vi "Expt 6.vi"() -> ()   [LabVIEW 2020]
panel:
  out "x >= 0?":bool
  out "current time":timestamp
  out "Y":dbl
  in  "y":dbl
  in  "x":dbl
  out "x2":dbl
  out "x1":dbl
  in  "c":dbl
  in  "b":dbl
  in  "a":dbl
  # "1)"
  # "2)"
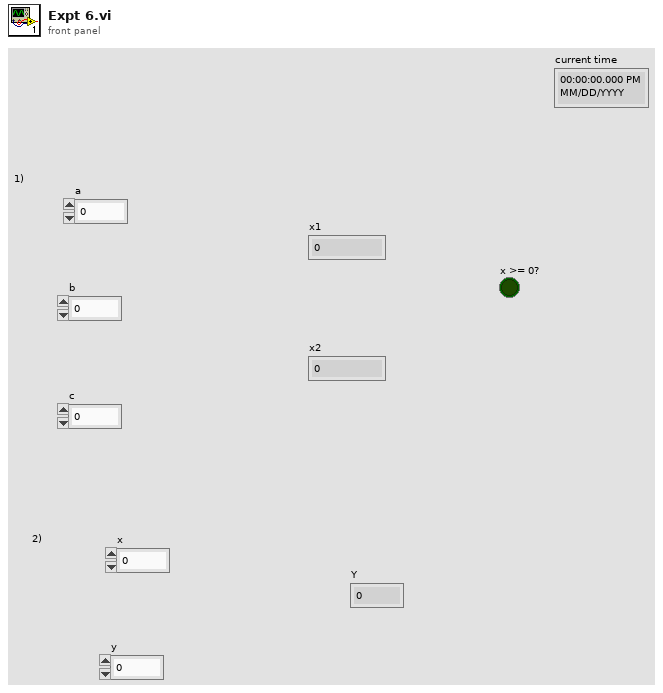
[diagram p1: front panel]
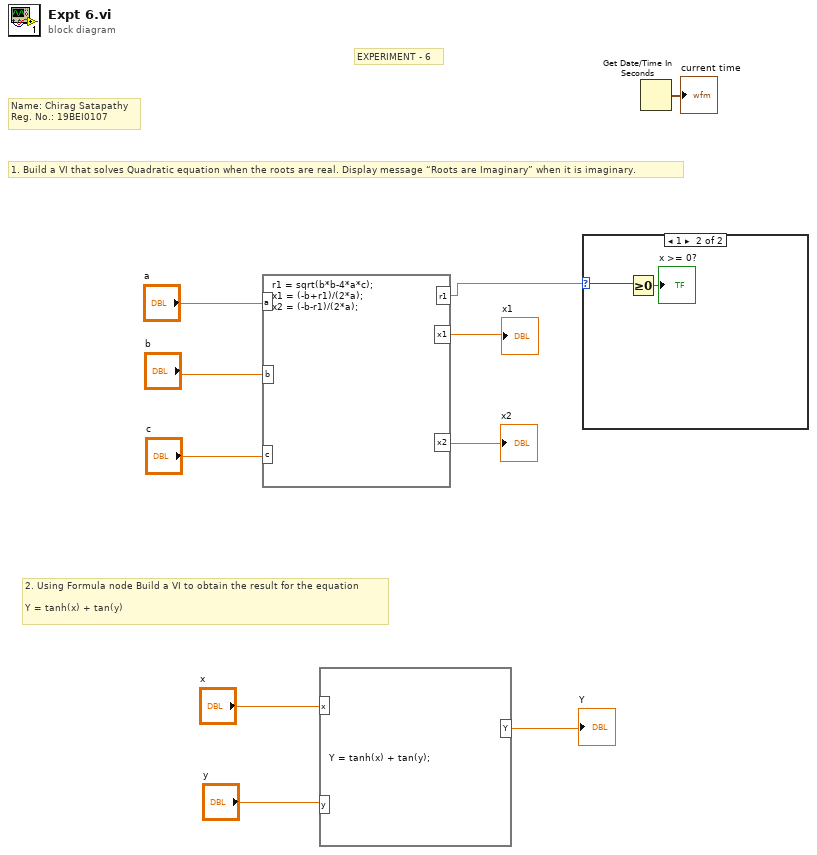
[diagram p0: block diagram]
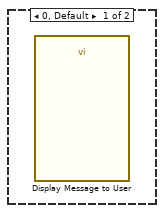
[diagram p2: hidden frame]
diagram:
  # "2. Using Formula node Build a VI to obtain the result for the equation\n\nY = tanh(x) + tan(y)"
  # "1. Build a VI that solves Quadratic equation when the roots are real. Display message “Roots are Imaginary” when it is imaginary."
  # "EXPERIMENT - 6"
  # "Name: Chirag Satapathy\nReg. No.: 19BEI0107"
  n1 = formula code="r1 = sqrt(b*b-4*a*c);\nx1 = (-b+r1)/(2*a);\nx2 = (-b-r1)/(2*a);"("a"="a", "b"="b", "c"="c") -> ("x1"=→"x1":dbl, "x2"=→"x2":dbl, "r1"=w1:dbl)
  n2 = formula code="Y = tanh(x) + tan(y);"("x"="x", "y"="y") -> ("Y"=→"Y":dbl)
  n3 = case shown="1" w1 {
    selector: w1 -> [_ w12]
    frame 0, Default {
      n4 = call "Display Message to User"() -> ()  [unwired: 10 in, 2 out]
    }
    frame 1 {
      n5 = Greater Or Equal To 0?(x=w12) -> (x >= 0?=→"x >= 0?":bool)
    }
  }
  n6 = Get Date/Time In Seconds() -> (seconds since 1Jan1904=→"current time":timestamp)
